vi "PI_WAV_line_dyn.vi"(5 "Attach to wav":bool, 7 "Axis Identifier":string, 8 "Amplitude / [mu]":dbl, 9 "Startpos / [mu]":dbl, 10 "Pixel per scan":u16, 11 "Commandset in":string[](array[string])) -> (1 "Curve-Start-Pixel":u16, 2 "Num_Pix":u16, 3 "Commandset out":string[](array[string]))   [LabVIEW 2011]
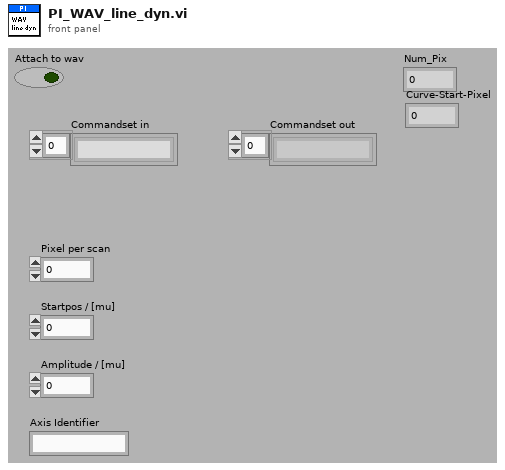
[diagram p1: front panel]
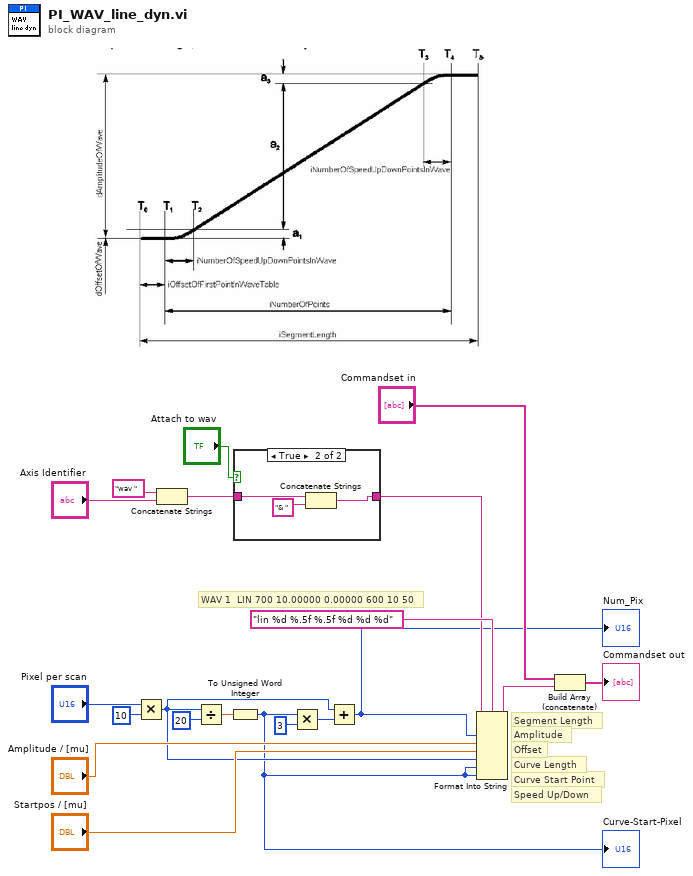
[diagram p0: block diagram]
diagram:
  # "Speed Up/Down"
  # "Curve Start Point"
  # "Curve Length"
  # "Offset"
  # "Amplitude"
  # "Segment Length"
  # "WAV 1  LIN 700 10.00000 0.00000 600 10 50"
  n1 = Multiply(x="Pixel per scan", y=u16 10) -> (x*y=w3:u16)
  n2 = Concatenate Strings("wav " ("new element/subarray"), "Axis Identifier") -> (w15:string)
  n3 = Divide(x=w3, y=u16 20) -> (x/y=w11:dbl)
  n4 = To Unsigned Word Integer(number=w11) -> (unsigned 16bit integer=w1:u16)
  "Curve-Start-Pixel" <- w1
  n5 = case shown="True" "Attach to wav" {
    tunnel: w15 -> [w21 w24]
    tunnel: [w21 w22] -> w7
    frame False {
    }
    frame True {
      n6 = Concatenate Strings(w24, "& " ("string")) -> (w22:string)
    }
  }
  n7 = Multiply(x=w1, y=u16 3) -> (x*y=w9:u16)
  n8 = Add(x=w3, y=w9) -> (x+y=w6:u16)
  "Num_Pix" <- w6
  n9 = Format Into String(format string="lin %d %.5f %.5f %d %d %d", initial string=w7, w6, "Amplitude / [mu]", "Startpos / [mu]", w3, w1, w1) -> (resulting string=w2:string)  [unwired: 1 in, 1 out]
  n10 = Build Array (concatenate)("Commandset in", w2) -> (→"Commandset out":string[])
